vi "SaveAs Document.vi"(8 "error in (no error)":errorcluster, 10 "Document Path":path, 11 "xwpfDocument in":refnum<class "xwpfDocument.lvclass">) -> (0 "error out":errorcluster, 3 "xwpfDocument out":refnum<class "xwpfDocument.lvclass">)   [LabVIEW 2017, in "Word_Specific.lvlib" / "xwpfDocument.lvclass"]
uses:
  xwpfDocument.lvclass
  xwpfDocument.lvclass/xwpfDocument.ctl
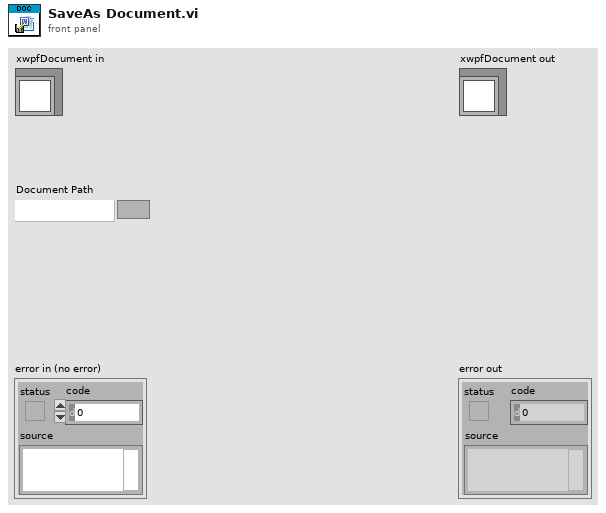
[diagram p1: front panel]
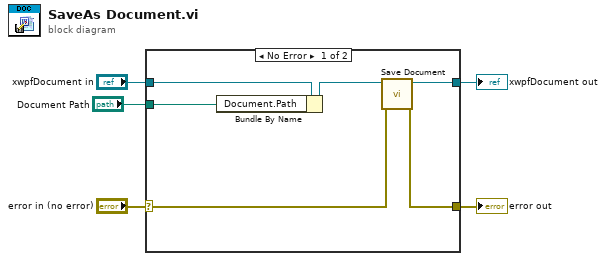
[diagram p0: block diagram]
diagram:
  n1 = case shown="No Error" "error in (no error)" {
    selector: "error in (no error)" -> [w10 w13]
    tunnel: [w8 w13] -> w4
    tunnel: [w9 w12] -> w2
    tunnel: "xwpfDocument in" -> [w11 w12]
    tunnel: "Document Path" -> [w6 _]
    frame No Error {
      n2 = Bundle By Name(cluster=w11, "Document.Path"=w6) -> (w7:refnum<class "xwpfDocument.lvclass">)
      n3 = call "Save Document.vi"("error in (no error)"=w10, "xwpfDocument in"=w7) -> ("error out"=w8:errorcluster, "xwpfDocument out"=w9:refnum<class "xwpfDocument.lvclass">)  [unwired: 8 in]
    }
    frame Error {
    }
  }
  "error out" <- w4
  "xwpfDocument out" <- w2
